vi "XYStage.isMoving.vi"(8 "error in (no error)":errorcluster, 11 "XYStage":refnum<class "XYStage.lvclass">) -> (0 "error out":errorcluster, 2 "Moving":bool, 3 "XYStage out":refnum<class "XYStage.lvclass">)   [LabVIEW 2015, in "XYStage.lvclass"]
doc: "---------------------------------------------------------------\nJKI State Machine Objects™\nhttp://jki.net/state-machine-objects/\nCopyright (C) 2005-2015, JKI <info@jki.net>\nALL RIGHTS RESERVEDJKI State Machine Objects (SMO) 1.0.0.4\nJKI - JKI\nCopyright (c) 2015, JKI"
uses:
  XYStage.lvclass
  Typedefs/(real)Coords--Cluster.ctl
panel:
  # "For instructions on how to use the JKI State Machine Objects, examples and video tutorials, visit:\nhttp://jki.net/state-machine-objects/\n\nJKI State Machine Objects™\nhttp://jki.net/state-machine-objects/\nCopyright (C) 2005-2015, JKI <info@jki.net>\nALL RIGHTS RESERVED"
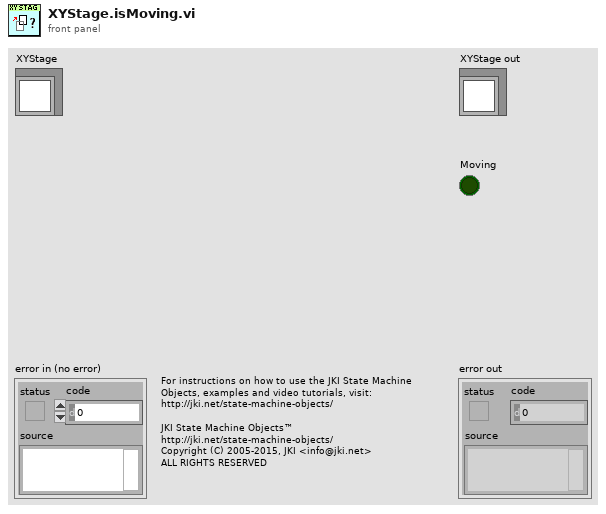
[diagram p1: front panel]
types:
  T1 = typedef "XYStage.lvclass/(real)Coords--Cluster.ctl" = cluster{"X":dbl, "Y":dbl}
  T2 = typedef "XYStage.lvclass/TargetPositions--Cluster.ctl" = cluster{"Coords":T1, "Counts":T3}
  T3 = typedef "XYStage.lvclass/(counts)Coords--Cluster.ctl" = cluster{"X":i32, "Y":i32}
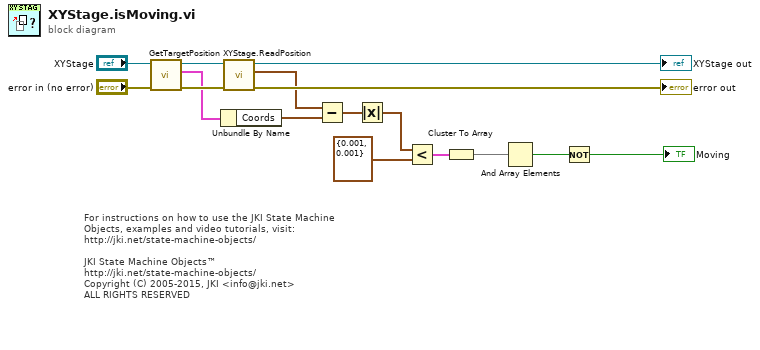
[diagram p0: block diagram]
diagram:
  # "For instructions on how to use the JKI State Machine Objects, examples and video tutorials, visit:\nhttp://jki.net/state-machine-objects/\n\nJKI State Machine Objects™\nhttp://jki.net/state-machine-objects/\nCopyright (C) 2005-2015, JKI <info@jki.net>\nALL RIGHTS RESERVED"
  n1 = call "GetTargetPosition.vi"("error in (no error)"="error in (no error)", "XYStage"="XYStage") -> ("error out"=w12:errorcluster, "Target"=w9:T2, "XYStage out"=w14:refnum<class "XYStage.lvclass">)  [unwired: 7 in]
  n2 = Unbundle By Name(w9) -> ("Coords"=w8:T1)
  n3 = call-dynamic "XYStage.ReadPosition.vi"("error in (no error)"=w12, "XYStage"=w14) -> ("error out"=→"error out":errorcluster, "Position"=w10:T1, "XYStage out"=→"XYStage out":refnum<class "XYStage.lvclass">)  [unwired: 6 in, 1 out]
  n4 = Subtract(x=w10, y=w8) -> (x-y=w7:T1)
  n5 = Absolute Value(x=w7) -> (abs(x)=w5:T1)
  n6 = Less?(x=w5, y=T1 {"X"=0.001, "Y"=0.001}) -> (x < y?=w4:cluster{"X":bool, "Y":bool})
  n7 = Cluster To Array(cluster=w4) -> (array=w3:bool[])
  n8 = And Array Elements(Boolean array=w3) -> (logical AND=w2:bool)
  n9 = Not(x=w2) -> (.not. x?=→"Moving":bool)
